vi "Graphics-Plot Colorbar.vi"(0 "Picture in":refnum<vi>, 2 "Map":T1(ring), 7 "Values":dbl[](array[numeric]), 11 "error in (no error)":errorcluster) -> (15 "error out":errorcluster)   [LabVIEW 2015]
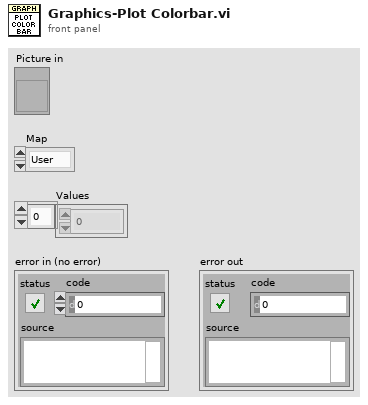
[diagram p1: front panel]
types:
  T1 = enum16{"User", "Prism", "Kelly", "Dark2", "Sequential", "Hue"}
  T2 = cluster{"left":i16, "top":i16, "right":i16, "bottom":i16}
  T3 = cluster{"horizontal":enum16{"left", "center", "right"}, "vertical":enum16{"top", "center", "bottom"}}
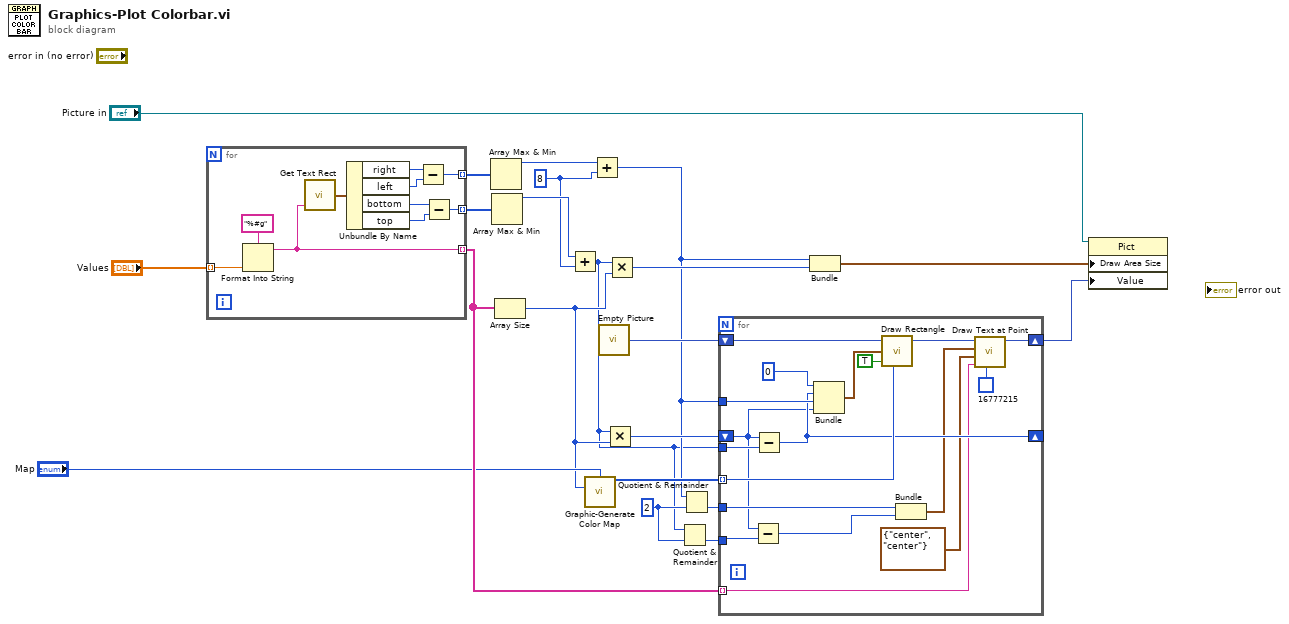
[diagram p0: block diagram]
diagram:
  w3 = i16 2 ("y")
  w8 = i16 8 ("y")
  n1 = for {
    tunnel: "Values" -> [w31] mode=indexing
    tunnel: [w30] -> w15 mode=indexing
    tunnel: [w25] -> w20 mode=indexing
    tunnel: [w22] -> w19 mode=indexing
    n2 = Format Into String(format string="%#g", w31) -> (resulting string=w30:string)  [unwired: 2 in, 1 out]
    n3 = call <vilib>:"Get Text Rect.vi"("text"=w30) -> ("rect"=w28:T2)  [unwired: 8 in]
    n4 = Unbundle By Name(w28) -> ("right"=w27:i16, "left"=w26:i16, "bottom"=w24:i16, "top"=w23:i16)
    n5 = Subtract(x=w27, y=w26) -> (x-y=w25:i16)
    n6 = Subtract(x=w24, y=w23) -> (x-y=w22:i16)
  }
  n7 = Array Max & Min(array=w20) -> (max value=w9:i16)  [unwired: 3 out]
  n8 = Array Max & Min(array=w19) -> (max value=w18:i16)  [unwired: 3 out]
  n9 = Array Size(array=w15) -> (size(s)=w7:i32)
  n10 = Add(x=w18, y=w8) -> (x+y=w2:i16)
  n11 = call "Graphic-Generate Color Map.vi"("Map"="Map", "Size"=w7) -> ("Colors"=w11:u32[])  [unwired: 13 in]
  n12 = Add(x=w9, y=w8) -> (x+y=w5:i16)
  n13 = call "Empty Picture"() -> ("empty picture"=w14:picture)
  n14 = Multiply(x=w2, y=w7) -> (x*y=w6:i32)
  n15 = Multiply(x=w2, y=w7) -> (x*y=w17:i32)
  n16 = Quotient & Remainder(x=w2, y=w3) -> (floor(x/y)=w1:i16)  [unwired: 1 out]
  n17 = Quotient & Remainder(x=w5, y=w3) -> (floor(x/y)=w4:i16)  [unwired: 1 out]
  n18 = for {
    tunnel: w15 -> [w38] mode=indexing
    tunnel: w2 -> [w49]
    shift-right: [w40] -> w13
    shift-left: w14 -> [w47]
    tunnel: w11 -> [w46] mode=indexing
    tunnel: w5 -> [w44]
    shift-right: [w42] -> _
    shift-left: w6 -> [w33]
    tunnel: w4 -> [w36]
    tunnel: w1 -> [w34]
    n19 = Subtract(x=w33, y=w34) -> (x-y=w32:i32)
    n20 = Subtract(x=w33, y=w49) -> (x-y=w42:i32)
    n21 = Bundle(0, w42, w44, w33) -> (w43:cluster{i32, i32, i16, i32})  [unwired: 1 in]
    n22 = call <vilib>:"Draw Rectangle.vi"("picture"=w47, "rect"=w43, "fill?(F)"=TRUE, "color(black)"=w46) -> ("new picture"=w41:picture)  [unwired: 5 in]
    n23 = Bundle(w36, w32) -> (w35:cluster{i16, i32})  [unwired: 1 in]
    n24 = call <vilib>:"Draw Text at Point.vi"("text color(black)"=u32 16777215, "text"=w38, "alignment(left, top)"=T3 {"horizontal"=enum."center", "vertical"=enum."center"}, "origin"=w35, "picture"=w41) -> ("new picture"=w40:picture)  [unwired: 5 in, 1 out]
  }
  n25 = Bundle(w5, w17) -> (w16:cluster{i16, i32})  [unwired: 1 in]
  n26 = property class="Pict"(reference="Picture in", "Draw Area Size"=w16, "Value"=w13) -> ()  [unwired: 1 in, 2 out]
